vi "Acquisition Message Loop.vi"(8 "error in (no error)":errorcluster, 9 "Data Queue":refnum<queue>, 10 "Data Notifier":refnum<notifier>, 11 "Message Queues":T1) -> (0 "error out":errorcluster)   [LabVIEW 2023, in "Acquisition.lvlib"]
doc: "Message loop for handling messages pertaining to the acquisition of data."
uses:
  Acquisition.lvlib
  support/Message Queue/All Message Queues.ctl
  support/Message Queue/Message Cluster.ctl
  Acquisition State.ctl
  support/Message Queue/Enqueue Message (Single).vi
  <vilib>/Utility/error.llb/Error Cluster From Error Code.vi
  <vilib>/ErrorRing/Error Ring.xnode
  support/Message Queue/Message Queue.lvlib
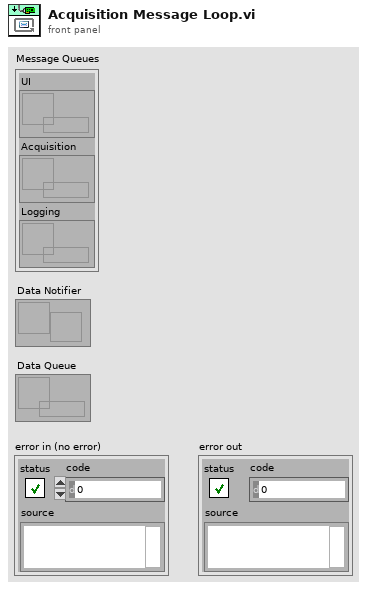
[diagram p1: front panel]
types:
  T1 = typedef "Message Queue.lvlib/All Message Queues.ctl" = cluster{"UI":refnum<queue>, "Acquisition":refnum<queue>, "Logging":refnum<queue>}
  T2 = typedef "Acquisition.lvlib/Acquisition State.ctl" = enum16{"Idle", "Acquiring"}
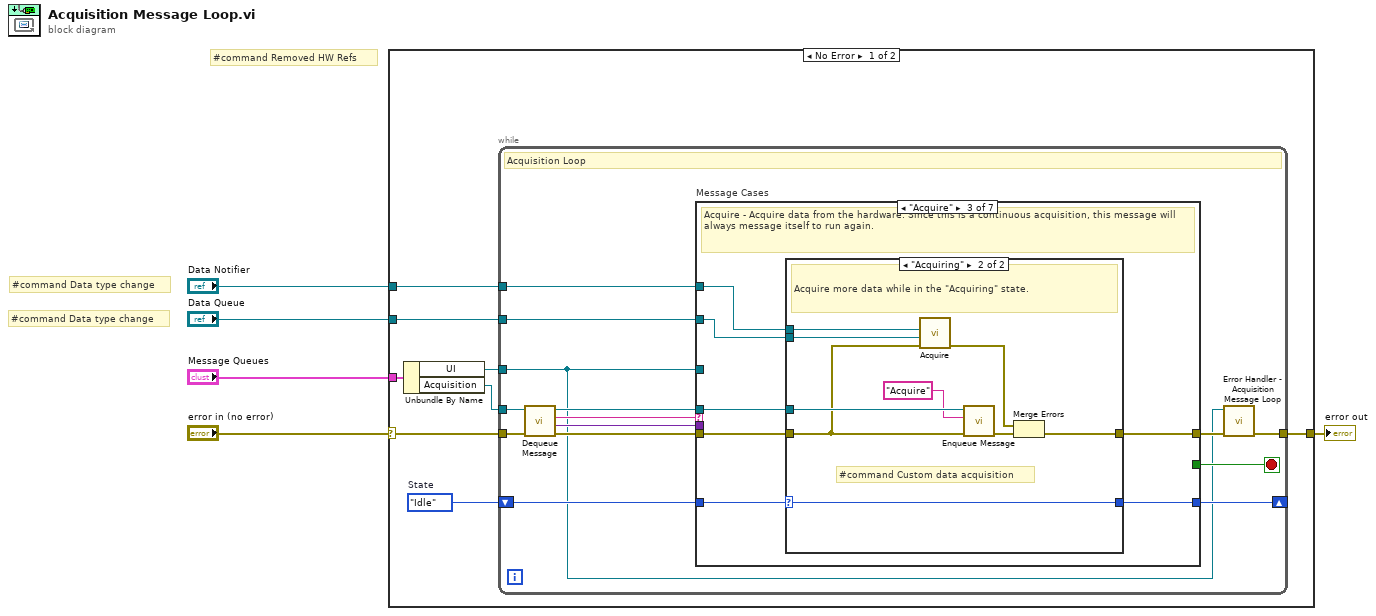
[diagram p0: block diagram]
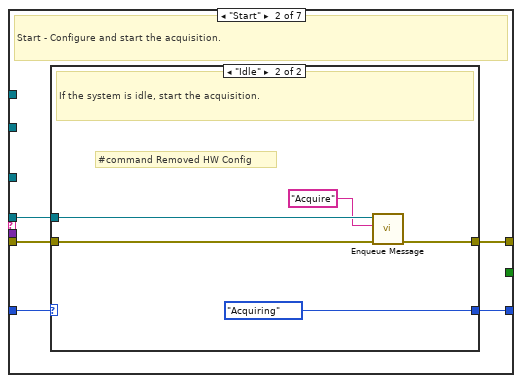
[diagram p3: hidden frame]
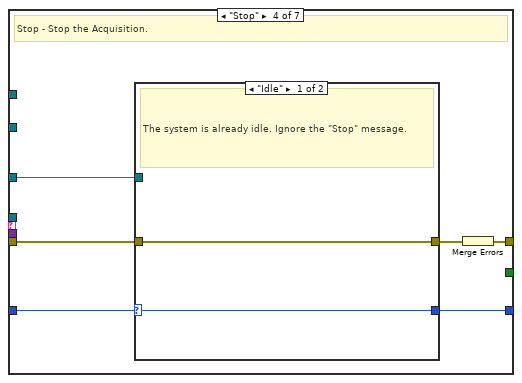
[diagram p6: hidden frame]
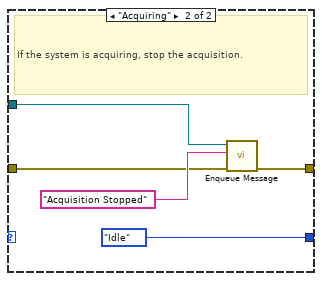
[diagram p7: hidden frame]
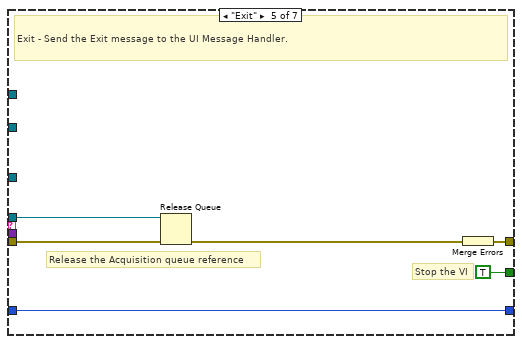
[diagram p8: hidden frame]
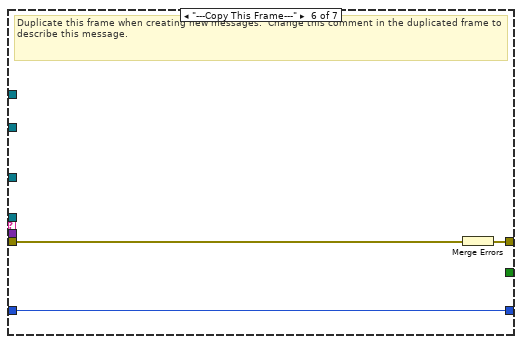
[diagram p9: hidden frame]
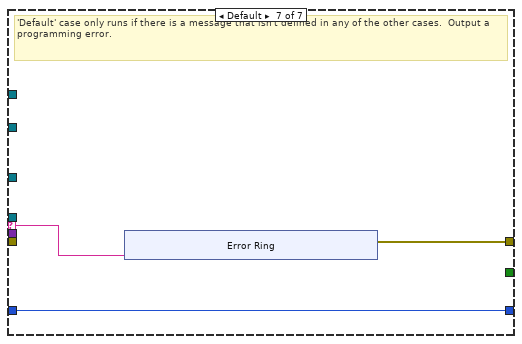
[diagram p10: hidden frame]
diagram:
  # "#command Removed HW Refs"
  # "#command Data type change"
  # "#command Data type change"
  n1 = case shown="No Error" "error in (no error)" {
    selector: "error in (no error)" -> [w10 w92]
    tunnel: "Message Queues" -> [w13 _]
    tunnel: [w11 w92] -> w4
    tunnel: "Data Notifier" -> [w8 _]
    tunnel: "Data Queue" -> [w7 _]
    frame No Error {
      w6 = Acquisition_State."Idle"  # State
      n2 = Unbundle By Name(w13) -> ("UI"=w9:refnum<queue>, "Acquisition"=w12:refnum<queue>)
      n3 = while {
        tunnel: w12 -> [w22]
        tunnel: w9 -> [w14]
        tunnel: w8 -> [w21]
        tunnel: w7 -> [w20]
        shift-right: [w18] -> _
        shift-left: w6 -> [w19]
        tunnel: w10 -> [w26]
        tunnel: [w17] -> w11
        stop <- w27 stop-if-true
        # "Acquisition Loop"
        n4 = call "Dequeue Message.vi"("error in (no error)"=w26, "Message Queue"=w22) -> ("error out"=w25:errorcluster, "Message Data"=w23:variant, "Message"=w24:string, "dup Message Queue"=w15:refnum<queue>)  [unwired: 6 in]
        n5 = case "Message Cases" shown="\"Acquire\"" w24 {
          selector: w24 -> [_ _ _ _ _ _ w82]
          tunnel: w15 -> [_ w32 w47 _ w74 _ _]
          tunnel: w25 -> [w29 w33 w46 w64 w76 w81 _]
          tunnel: [w29 w34 w48 w65 w77 w80 w83] -> w16
          tunnel: [_ _ _ _ TRUE _ _] -> w27
          tunnel: w23 -> [_ _ _ _ _ _ _]
          tunnel: w14 -> [_ _ _ w60 _ _ _]
          tunnel: w21 -> [_ _ w45 _ _ _ _]
          tunnel: w20 -> [_ _ w44 _ _ _ _]
          tunnel: w19 -> [w28 w30 w42 w62 w73 w79 w84]
          tunnel: [w28 w31 w43 w61 w73 w79 w84] -> w18
          frame "Initialize" {
            # "Initialize  - Initialize is currently a no-op.  The hardware initialization takes place in the 'Start' message."
          }
          frame "Start" {
            # "Start - Configure and start the acquisition."
            n6 = case shown="\"Idle\"" w30 {
              selector: w30 -> [w35 _]
              tunnel: [w36 w37] -> w34
              tunnel: w33 -> [w36 w41]
              tunnel: w32 -> [_ w40]
              tunnel: [w35 Acquisition_State."Acquiring" ("Acquisition State")] -> w31
              frame "Acquiring" {
                # "The system is already acquiring. Ignore the \"Start\" message."
              }
              frame "Idle" {
                # "#command Removed HW Config"
                # "If the system is idle, start the acquisition."
                n7 = call-poly "Enqueue Message.vi"("error in (no error)"=w41, "Message"="Acquire", "Message Queue"=w40) -> ("error out"=w37:errorcluster)  [unwired: 7 in, 1 out]
              }
            }
          }
          frame "Acquire" {
            # "Acquire - Acquire data from the hardware. Since this is a continuous acquisition, this message will always message itself to run again."
            n8 = case shown="\"Acquiring\"" w42 {
              selector: w42 -> [w49 w52]
              tunnel: [w50 w59] -> w48
              tunnel: w47 -> [_ w57]
              tunnel: w46 -> [w50 w51]
              tunnel: w45 -> [_ w54]
              tunnel: w44 -> [_ w53]
              tunnel: [w49 w52] -> w43
              frame "Idle" {
                # "Ignore \"Acquire\" messages when the acquisition is idle."
              }
              frame "Acquiring" {
                # "#command Custom data acquisition"
                # "Acquire more data while in the \"Acquiring\" state."
                n9 = call "Acquire.vi"("error in (no error)"=w51, "Data Queue"=w53, "Data Notifier"=w54) -> ("error out"=w56:errorcluster)  [unwired: 8 in]
                n10 = call-poly "Enqueue Message.vi"("error in (no error)"=w51, "Message"="Acquire", "Message Queue"=w57) -> ("error out"=w58:errorcluster)  [unwired: 7 in, 1 out]
                n11 = Merge Errors(w56, w58) -> (w59:errorcluster)
              }
            }
          }
          frame "Stop" {
            # "Stop - Stop the Acquisition."
            n12 = case shown="\"Idle\"" w62 {
              selector: w62 -> [w66 _]
              tunnel: w64 -> [w67 w68]
              tunnel: [w67 w71] -> w63
              tunnel: [w66 Acquisition_State."Idle" ("State")] -> w61
              tunnel: w60 -> [_ w70]
              frame "Idle" {
                # "The system is already idle. Ignore the \"Stop\" message."
              }
              frame "Acquiring" {
                # "If the system is acquiring, stop the acquisition."
                n13 = call-poly "Enqueue Message.vi"("error in (no error)"=w68, "Message"="Acquisition Stopped", "Message Queue"=w70) -> ("error out"=w71:errorcluster)  [unwired: 7 in, 1 out]
              }
            }
            n14 = Merge Errors(w63) -> (w65:errorcluster)
          }
          frame "Exit" {
            # "Release the Acquisition queue reference"
            # "Stop the VI"
            # "Exit - Send the Exit message to the UI Message Handler."
            n15 = Release Queue(queue=w74, error in (no error)=w76) -> (error out=w75:errorcluster)  [unwired: 1 in, 2 out]
            n16 = Merge Errors(w75) -> (w77:errorcluster)
          }
          frame "---Copy This Frame---" {
            # "Duplicate this frame when creating new messages.  Change this comment in the duplicated frame to describe this message."
            n17 = Merge Errors(w81) -> (w80:errorcluster)
          }
          frame Default {
            # "'Default' case only runs if there is a message that isn't defined in any of the other cases.  Output a programming error."
            n18 = xnode "Error Ring"("parameter 0"=w82) -> ("error out"=w83:errorcluster)
          }
        }
        n19 = call "Error Handler - Acquisition Message Loop.vi"("error in (no error)"=w16, "Message Queue"=w14) -> ("dup error in"=w17:errorcluster)  [unwired: 8 in, 1 out]
      }
    }
    frame Error {
    }
  }
  "error out" <- w4
